vi "Read DAQmxTask dict-mem.vi"(8 "error in (no error)":errorcluster, 10 "Task name":T1, 11 "Control in":refnum<class "Control.lvclass">) -> (0 "error out":errorcluster, 2 "DAQmx task class":refnum<class "DAQmxTask.lvclass">, 3 "Control out":refnum<class "Control.lvclass">)   [LabVIEW 2015, in "Control.lvclass"]
uses:
  Control.lvclass
  dependecies/ControlsVIs/Clusters-def/list-of-DAQmx-tasks.ctl
  DAQmxTasks/DAQmxTask.lvclass
  Control.lvclass/Control.ctl
  DAQmxTasks/DAQmxTasklDInput/DAQmxTaskDInput.lvclass
  DAQmxTasks/DAQmxTaskAICurrent.lvclass
  DAQmxTasks/DAQmxTaskDOutput/DAQmxTaskDOutput.lvclass
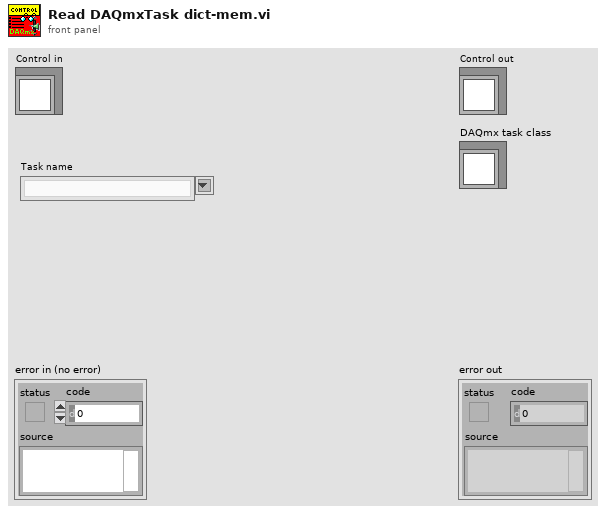
[diagram p1: front panel]
types:
  T1 = typedef "list-of-DAQmx-tasks.ctl" = string
  T2 = cluster{"class name":string, "DAQmxTask.lvclass":refnum<class "DAQmxTask.lvclass">}
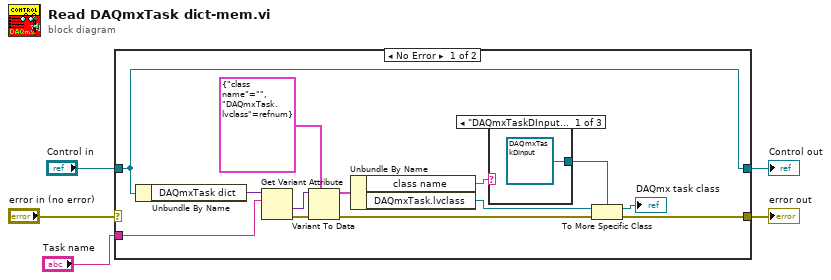
[diagram p0: block diagram]
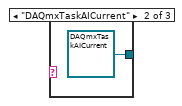
[diagram p2: hidden frame]
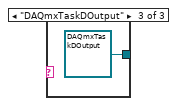
[diagram p3: hidden frame]
diagram:
  n1 = case shown="No Error" "error in (no error)" {
    selector: "error in (no error)" -> [_ w22]
    tunnel: [w7 w22] -> w4
    tunnel: [w18 w23] -> w2
    tunnel: "Control in" -> [w18 w23]
    tunnel: "Task name" -> [w14 _]
    frame No Error {
      n2 = Unbundle By Name(w18) -> ("DAQmxTask dict"=w17:variant)
      n3 = Get Variant Attribute(Variant=w17, name=w14) -> (value=w15:variant, error out=w16:errorcluster)  [unwired: 2 in, 2 out]
      n4 = Variant To Data(error in=w16, type=T2 {"class name"="", "DAQmxTask.lvclass"=refnum} ("input cluster"), Variant=w15) -> (data=w12:T2, error out=w8:errorcluster)
      n5 = Unbundle By Name(w12) -> ("class name"=w11:string, "DAQmxTask.lvclass"=w9:refnum<class "DAQmxTask.lvclass">)
      n6 = case shown="\"DAQmxTaskDInput\", Default" w11 {
        tunnel: [refnum<class "DAQmxTaskDInput.lvclass"> refnum ("DAQmxTaskDInput.lvclass") refnum<class "DAQmxTaskAICurrent.lvclass"> refnum ("DAQmxTaskAICurrent.lvclass") refnum<class "DAQmxTaskDOutput.lvclass"> refnum ("DAQmxTaskDOutput.lvclass")] -> w10
        frame "DAQmxTaskDInput", Default {
        }
        frame "DAQmxTaskAICurrent" {
        }
        frame "DAQmxTaskDOutput" {
        }
      }
      n7 = To More Specific Class(target class=w10, reference=w9, error in=w8) -> (specific class reference=→"DAQmx task class":refnum<class "DAQmxTask.lvclass">, error out=w7:errorcluster)
    }
    frame Error {
    }
  }
  "error out" <- w4
  "Control out" <- w2
